vi "10_jak_zasilat_frontou_ruzne_datove_typy.vi"() -> ()   [LabVIEW 2019]
panel:
  out "Waveform Chart 3":dbl(graph)
  out "Waveform Chart 2":dbl(graph)
  out "Cas":timestamp
  out "x = 0?":bool
  out "Waveform Chart":dbl(graph)
  in  "stop":bool
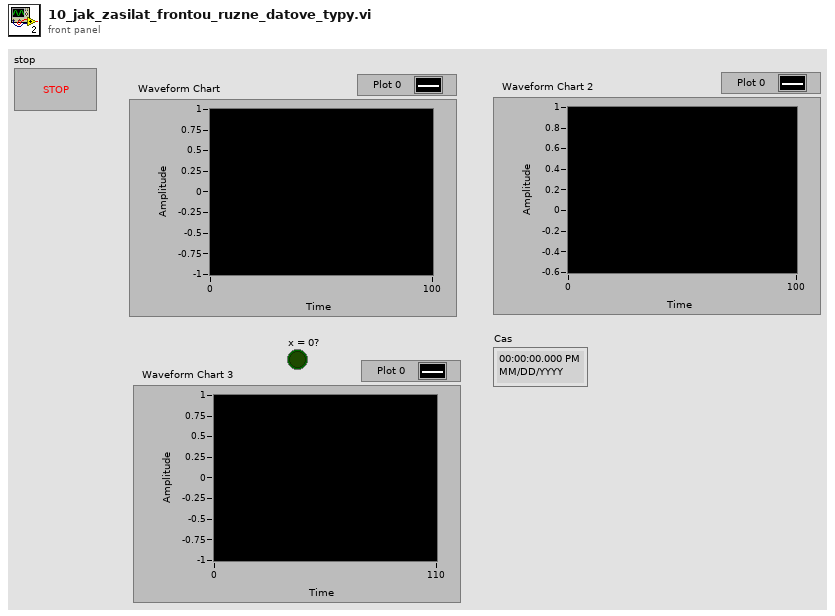
[diagram p1: front panel]
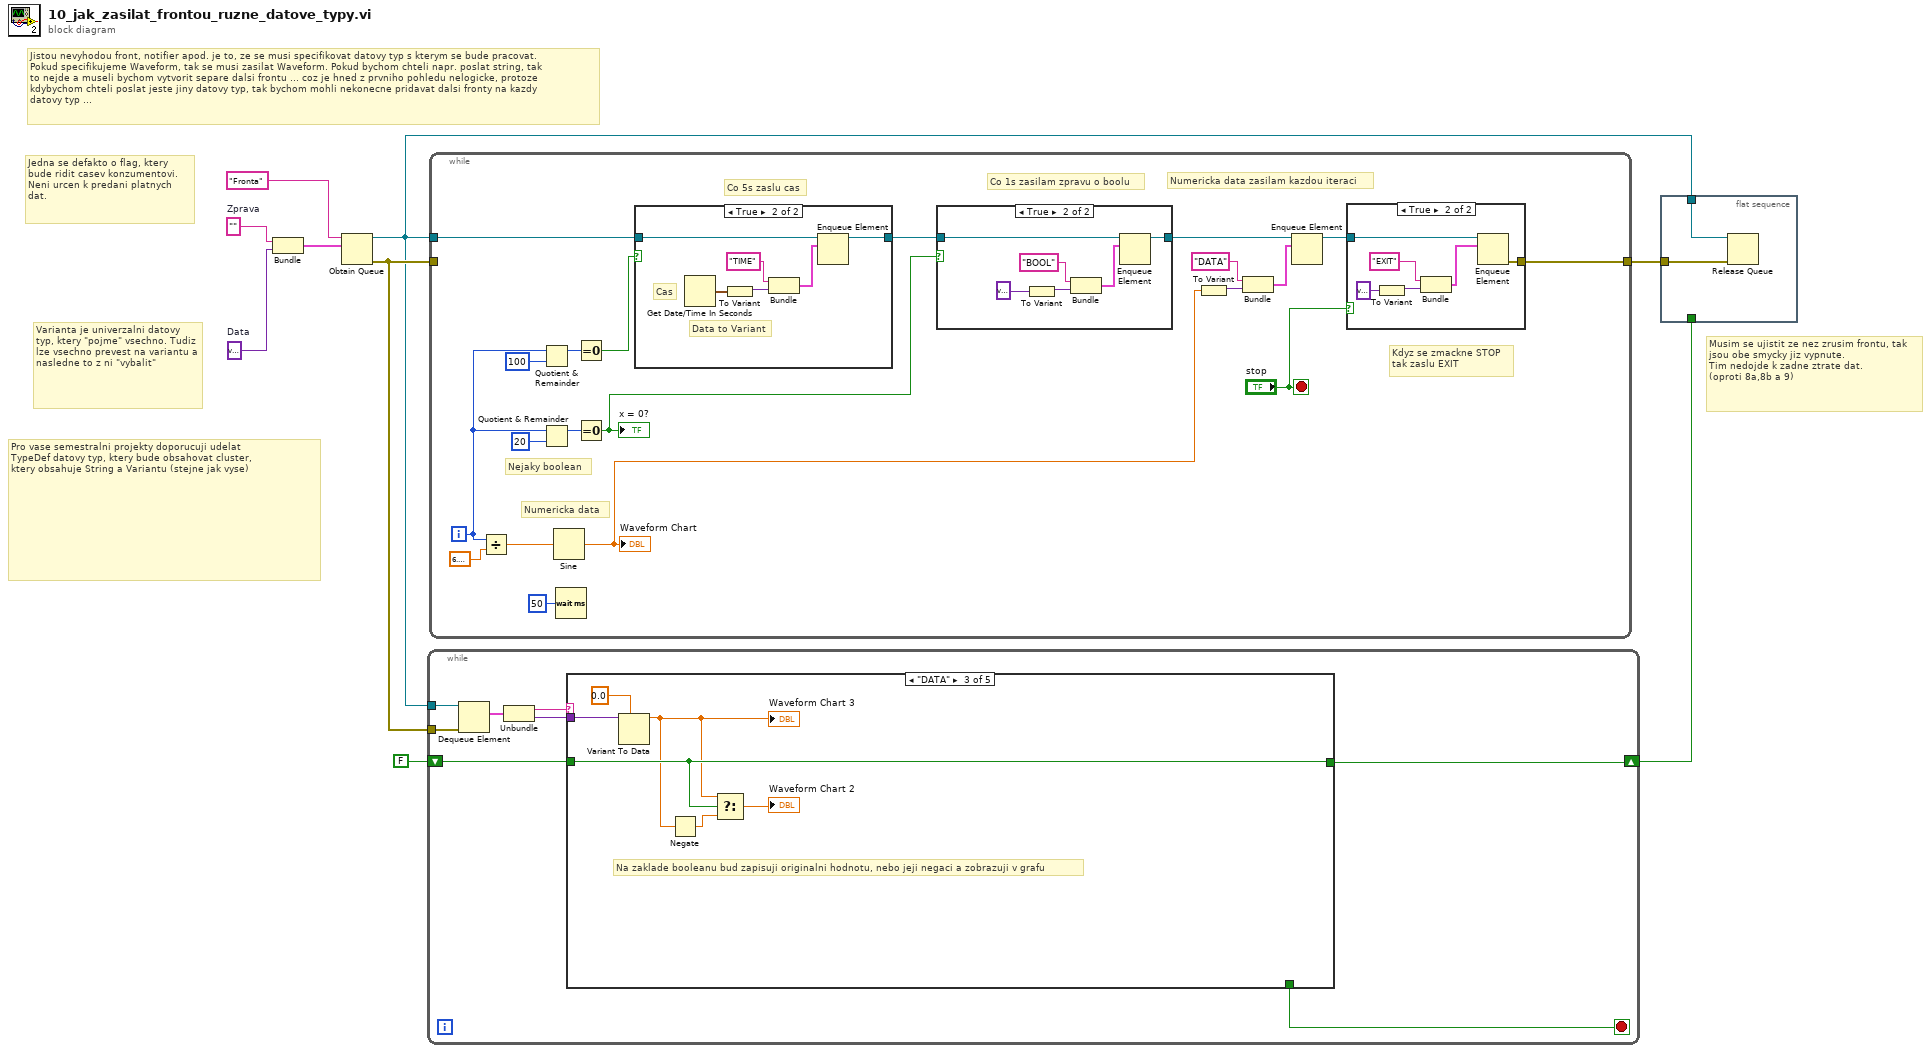
[diagram p0: block diagram]
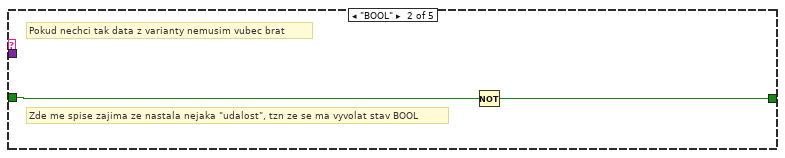
[diagram p3: hidden frame]
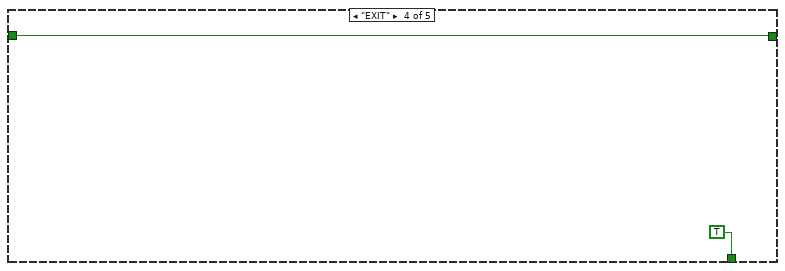
[diagram p4: hidden frame]
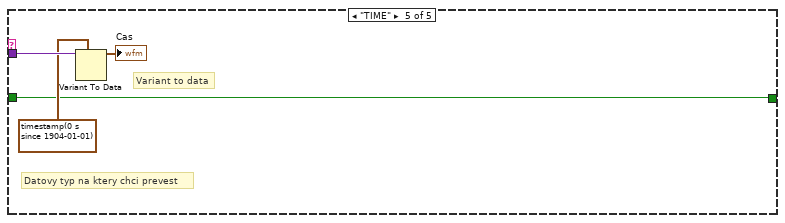
[diagram p5: hidden frame]
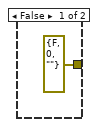
[diagram p6: hidden frame]
diagram:
  w8 = variant  # Data
  w9 = ""  # Zprava
  # "Pro vase semestralni projekty doporucuji udelat\nTypeDef datovy typ, ktery bude obsahovat cluster,\nktery obsahuje String a Variantu (stejne jak vyse)"
  # "Musim se ujistit ze nez zrusim frontu, tak jsou obe smycky jiz vypnute.\nTim nedojde k zadne ztrate dat.\n(oproti 8a,8b a 9)"
  # "Varianta je univerzalni datovy typ, ktery \"pojme\" vsechno. Tudiz lze vsechno prevest na variantu a nasledne to z ni \"vybalit\""
  # "Jedna se defakto o flag, ktery bude ridit casev konzumentovi.\nNeni urcen k predani platnych dat."
  # "Jistou nevyhodou front, notifier apod. je to, ze se musi specifikovat datovy typ s kterym se bude pracovat.\nPokud specifikujeme Waveform, tak se musi zasilat Waveform. Pokud bychom chteli napr. poslat string, tak \nto nejde a museli bychom vytvorit separe dalsi frontu ... coz je hned z prvniho pohledu nelogicke, protoze\nkdybychom chteli poslat jeste jiny datovy typ, tak bychom mohli nekonecne pridavat dalsi fronty na kazdy \ndatovy typ ..."
  n1 = Bundle("Zprava"=w9, "Data"=w8) -> (w7:cluster{"Zprava":string, "Data":variant})  [unwired: 1 in]
  n2 = Obtain Queue(name (unnamed)="Fronta", element data type=w7) -> (queue out=w3:refnum<queue>, error out=w5:errorcluster)  [unwired: 3 in, 1 out]
  n3 = while {
    tunnel: w3 -> [w16]
    tunnel: w5 -> [w17]
    shift-right: [w11] -> w1
    shift-left: FALSE -> [w12]
    stop <- w10 stop-if-true
    n4 = Dequeue Element(queue=w16, error in (no error)=w17) -> (element=w15:cluster{"Zprava":string, "Data":variant})  [unwired: 1 in, 3 out]
    n5 = Unbundle(w15) -> ("Zprava"=w14:string, "Data"=w13:variant)
    n6 = case shown="\"DATA\"" w14 {
      tunnel: w13 -> [_ _ w26 _ w32]
      tunnel: w12 -> [w18 w20 w24 w28 w29]
      tunnel: [w18 w19 w24 w28 w29] -> w11
      tunnel: [_ _ _ TRUE _] -> w10
      frame "False", Default {
      }
      frame "BOOL" {
        # "Zde me spise zajima ze nastala nejaka \"udalost\", tzn ze se ma vyvolat stav BOOL"
        # "Pokud nechci tak data z varianty nemusim vubec brat"
        n7 = Not(x=w20) -> (.not. x?=w19:bool)
      }
      frame "DATA" {
        # "Na zaklade booleanu bud zapisuji originalni hodnotu, nebo jeji negaci a zobrazuji v grafu"
        n8 = Variant To Data(type=0.0, Variant=w26) -> (data=w21:dbl)  [unwired: 1 in, 1 out]
        "Waveform Chart 3" <- w21
        n9 = Negate(x=w21) -> (-x=w23:dbl)
        n10 = Select(t=w21, s=w24, f=w23) -> (s? t:f=→"Waveform Chart 2":dbl)
      }
      frame "EXIT" {
      }
      frame "TIME" {
        # "Variant to data"
        # "Datovy typ na ktery chci prevest"
        n11 = Variant To Data(type=timestamp(0 s since 1904-01-01), Variant=w32) -> (data=→"Cas":timestamp)  [unwired: 1 in, 1 out]
      }
    }
  }
  n12 = while {
    tunnel: w3 -> [w47]
    tunnel: w5 -> [_]
    tunnel: [w33] -> w2
    i -> [w44]
    stop <- "stop" stop-if-true
    # "Kdyz se zmackne STOP\ntak zaslu EXIT"
    # "Numericka data zasilam kazdou iteraci"
    # "Co 1s zasilam zpravu o boolu"
    # "Co 5s zaslu cas"
    # "Nejaky boolean"
    # "Numericka data"
    n13 = Divide(x=w44, y=6.283185307179586) -> (x/y=w50:dbl)
    n14 = Quotient & Remainder(x=w44, y=100) -> (x-y*floor(x/y)=w46:i32)  [unwired: 1 out]
    n15 = Quotient & Remainder(x=w44, y=20) -> (x-y*floor(x/y)=w48:i32)  [unwired: 1 out]
    n16 = Sine(x=w50) -> (sin(x)=w36:dbl)
    "Waveform Chart" <- w36
    n17 = Wait (ms)(milliseconds to wait=u32 50) -> ()  [unwired: 1 out]
    n18 = Equal To 0?(x=w46) -> (x = 0?=w43:bool)
    n19 = Equal To 0?(x=w48) -> (x = 0?=w41:bool)
    "x = 0?" <- w41
    n20 = case shown="True" w43 {
      tunnel: w47 -> [w67 w73]
      tunnel: [w67 w68] -> w42
      frame False {
      }
      frame True {
        # "Data to Variant"
        # "Cas"
        n21 = Get Date/Time In Seconds() -> (seconds since 1Jan1904=w71:timestamp)
        n22 = To Variant(anything=w71) -> (Variant=w70:variant)
        n23 = Bundle("TIME", "Variant"=w70) -> (w69:cluster{string, "Variant":variant})  [unwired: 1 in]
        n24 = Enqueue Element(queue=w73, element=w69) -> (queue out=w68:refnum<queue>)  [unwired: 2 in, 2 out]
      }
    }
    n25 = case shown="True" w41 {
      tunnel: w42 -> [w60 w66]
      tunnel: [w60 w61] -> w40
      frame False {
      }
      frame True {
        n26 = To Variant(anything=variant) -> (Variant=w64:variant)
        n27 = Bundle("BOOL", "Variant"=w64) -> (w63:cluster{string, "Variant":variant})  [unwired: 1 in]
        n28 = Enqueue Element(queue=w66, element=w63) -> (queue out=w61:refnum<queue>)  [unwired: 2 in, 2 out]
      }
    }
    n29 = To Variant(anything=w36) -> (Variant=w38:variant)
    n30 = Bundle("DATA", "Variant"=w38) -> (w37:cluster{string, "Variant":variant})  [unwired: 1 in]
    n31 = Enqueue Element(queue=w40, element=w37) -> (queue out=w35:refnum<queue>)  [unwired: 2 in, 2 out]
    n32 = case shown="True" "stop" {
      tunnel: w35 -> [_ w56]
      tunnel: [errorcluster {"status"=FALSE, "code"=0, "source"=""} ("error out") w54] -> w33
      frame False {
      }
      frame True {
        n33 = To Variant(anything=variant) -> (Variant=w58:variant)
        n34 = Bundle("EXIT", "Variant"=w58) -> (w59:cluster{string, "Variant":variant})  [unwired: 1 in]
        n35 = Enqueue Element(queue=w56, element=w59) -> (error out=w54:errorcluster)  [unwired: 2 in, 2 out]
      }
    }
  }
  n36 = flat-sequence {
    tunnel: w3 -> [w75]
    tunnel: w2 -> [w74]
    tunnel: w1 -> [_]
    frame #0 {
      n37 = Release Queue(queue=w75, error in (no error)=w74) -> ()  [unwired: 1 in, 3 out]
    }
  }
